vi "Get Required Aliases for Multi Instrument Msg.vi"(8 "error in (no error)":errorcluster, 10 "Alias Table in":variant, 11 "Multi Instrument Msg in":refnum<class "Multi Instrument Msg.lvclass">) -> (0 "error out":errorcluster, 1 "Alias Sub Table":variant, 2 "Alias Table out":variant, 3 "Multi Instrument Msg out":refnum<class "Multi Instrument Msg.lvclass">, 4 "Alias Array":string[](array[string]), 5 "All Instruments Present?":bool)   [LabVIEW 2020, in "Instrument Handler.lvlib" / "Instrument Handler.lvclass"]
doc: "Get all instruments aliases required for the execution of a Multi Instrument Msg from the Alias Table. The found aliases are returned as a string array and in an Alias Sub Table."
uses:
  Instrument Handler.lvclass
  Messages/Multi Instrument Msg/Multi Instrument Msg.lvclass
  PPL/HDH.Data.Generic.lvlibp
  PPL/HDH.Actor Framework.Core.Instrument Driver.lvlibp/Instrument Driver/Instrument Driver.lvclass
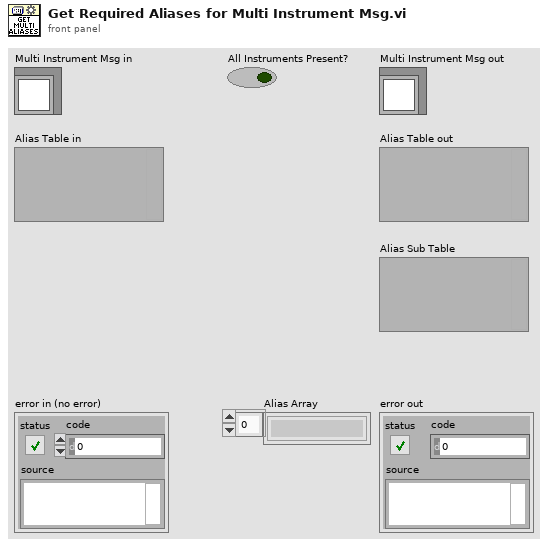
[diagram p1: front panel]
types:
  T1 = typedef "Instrument Handler.lvlib/Multi Instrument Msg.lvclass/Ctl_RequiredInstrumentElement.ctl" = cluster{"Count":i16, "Driver":refnum<class "Instrument Driver.lvclass">}
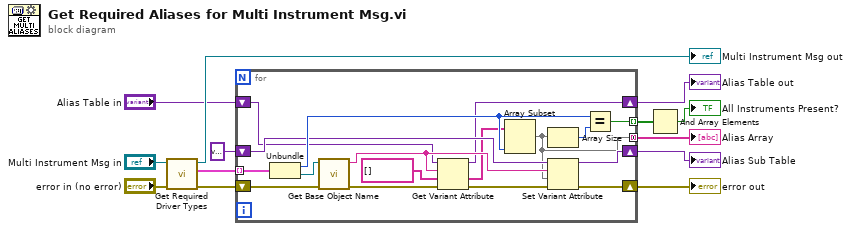
[diagram p0: block diagram]
diagram:
  n1 = call-dynamic "Get Required Driver Types.vi"("error in (no error)"="error in (no error)", "Multi Instrument Msg in"="Multi Instrument Msg in") -> ("error out"=w13:errorcluster, "Required Driver Types"=w11:T1[], "Multi Instrument Msg out"=→"Multi Instrument Msg out":refnum<class "Multi Instrument Msg.lvclass">)  [unwired: 7 in]
  n2 = for {
    tunnel: w11 -> [w30] mode=indexing
    tunnel: [w17] -> w3 mode=concatenating
    tunnel: [w24] -> w1 mode=indexing
    shift-right: [w18] -> w4
    shift-left: w13 -> [w28]
    shift-right: [w22] -> w6
    shift-left: variant -> [w23]
    shift-right: [w15] -> w8
    shift-left: "Alias Table in" -> [w16]
    n3 = Unbundle(w30) -> ("Count"=w25:i16, "Driver"=w29:refnum<class "Instrument Driver.lvclass">)
    n4 = call "Get Base Object Name.vi"("error in (no error)"=w28, "Object in"=w29) -> ("error out"=w27:errorcluster, "Base class name"=w21:string)  [unwired: 8 in]
    n5 = Get Variant Attribute(Variant=w16, name=w21, default value (empty Variant)=string[] [] ("Base class name"), error in=w27) -> (duplicate Variant=w15:variant, value=w20:string[], error out=w19:errorcluster)  [unwired: 1 out]
    n6 = Array Subset(array=w20, length=w25) -> (w17:string[])  [unwired: 1 in]
    n7 = Array Size(array=w17) -> (size(s)=w26:i32)
    n8 = Set Variant Attribute(Variant=w23, name=w21, value=w17, error in=w19) -> (Variant out=w22:variant, error out=w18:errorcluster)  [unwired: 1 out]
    n9 = Equal?(x=w25, y=w26) -> (x = y?=w24:bool)
  }
  "Alias Table out" <- w8
  "Alias Sub Table" <- w6
  "error out" <- w4
  "Alias Array" <- w3
  n10 = And Array Elements(Boolean array=w1) -> (logical AND=→"All Instruments Present?":bool)
